vi "Sinusoidal Stop.vi"(8 "error in (no error)":errorcluster, 9 "Device and Axis":string, 11 "VISA resource name":refnum<visa-resource-name>) -> (0 "error out":errorcluster, 3 "VISA resource name out":refnum<visa-resource-name>)   [LabVIEW 2015, in "Zaber A Series.lvlib"]
doc: "Halts a sinusoidal motion already in progress at the next cycle boundary.\n\nThe normal stop command (see the Stop VI) will decelerate a sinusoidal motion immediately. Use this sinusoidal stop command if you want motion to halt after a whole number of cycles.\n\nThis VI requires that the Initialize VI has been called with the same serial port."
uses:
  Zaber A Series.lvlib
  Private/All Commands.ctl
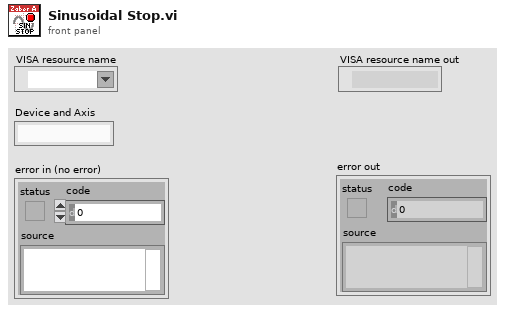
[diagram p1: front panel]
types:
  T1 = typedef "Zaber A Series.lvlib/All Commands.ctl" = string
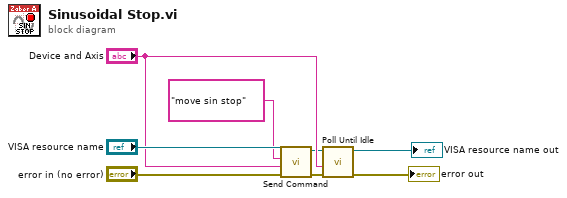
[diagram p0: block diagram]
diagram:
  n1 = call "Send Command.vi"("error in (no error)"="error in (no error)", "Device and Axis"="Device and Axis", "Command"=T1 "move sin stop" ("Command List"), "VISA resource name"="VISA resource name") -> ("error out"=w5:errorcluster, "VISA resource name out"=w4:refnum<visa-resource-name>)  [unwired: 2 in, 4 out]
  n2 = call "Poll Until Idle.vi"("error in (no error)"=w5, "Device and Axis"="Device and Axis", "VISA resource name"=w4) -> ("error out"=→"error out":errorcluster, "VISA resource name out"=→"VISA resource name out":refnum<visa-resource-name>)  [unwired: 7 in]
